vi "Find Ruby.vi"(8 "Error In":errorcluster) -> (0 "Error Out":errorcluster, 2 "Names":string[](array[string]), 3 "Recorders List":refnum<class "Instrument Actor.lvclass">[](array[class]))   [LabVIEW 2016, in "Ruby Spectra.lvclass"]
uses:
  Ruby Spectra.lvclass
  Instrument Actor/Instrument Actor.lvclass
  C:/github/LabActor/Recorders/Spectrometer/Spectrometer.lvclass
  C:/github/LabActor/Instrument Actor/Instrument Actor.lvclass
  NHMFL_Core/Libraries/Instruments/Ocean Optics/Ocean Optics Driver/Ocean Optics Driver.lvclass
  C:/github/NHMFL_Core/Libraries/Instruments/VISA Instrument/VISA Instrument.lvclass
  C:/github/NHMFL_Core/Libraries/Instruments/Spectrometer Driver/Spectrometer Driver.lvclass
  NHMFL_Core/Libraries/Instruments/VISA Instrument/VISA Instrument.lvclass/VISA Instrument.ctl
  NHMFL_Core/Libraries/Instruments/VISA Instrument/Write VISA resource.vi
  Spectrometer/Write Spectrometer Driver.lvclass.vi
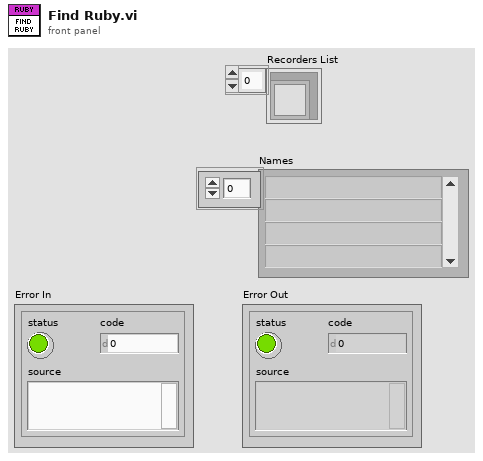
[diagram p1: front panel]
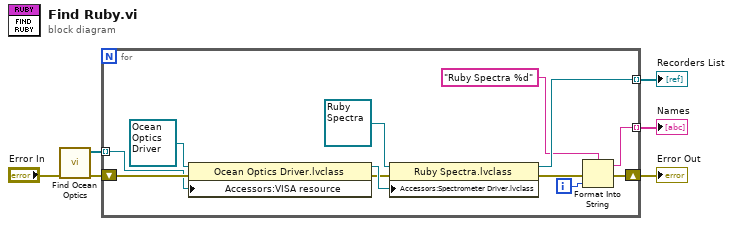
[diagram p0: block diagram]
diagram:
  n1 = call "Find Ocean Optics.vi"("Error In"="Error In") -> ("Error Out"=w4:errorcluster, "Devices"=w5:refnum<visa-resource-name>[])  [unwired: 9 in]
  n2 = for {
    tunnel: w5 -> [w13] mode=indexing
    shift-right: [w9] -> w3
    shift-left: w4 -> [w14]
    tunnel: [w12] -> w2 mode=indexing
    tunnel: [w8] -> w1 mode=indexing
    i -> [w11]
    n3 = property class="Ocean Optics Driver.lvclass"(reference=refnum<class "Ocean Optics Driver.lvclass"> refnum ("Ocean Optics Driver.lvclass"), error in=w14, "Accessors:VISA resource"=w13) -> (reference out=w18:refnum<class "Ocean Optics Driver.lvclass">, error out=w16:errorcluster)
    n4 = property class="Ruby Spectra.lvclass"(reference=refnum<class "Ruby Spectra.lvclass"> refnum ("Ruby Spectra.lvclass"), error in=w16, "Accessors:Spectrometer Driver.lvclass"=w18) -> (reference out=w8:refnum<class "Ruby Spectra.lvclass">, error out=w10:errorcluster)
    n5 = Format Into String(format string="Ruby Spectra %d", error in=w10, w11) -> (resulting string=w12:string, error out=w9:errorcluster)  [unwired: 1 in]
  }
  "Error Out" <- w3
  "Recorders List" <- w1
  "Names" <- w2
